vi "BMS.vi"() -> ()   [LabVIEW 2016]
panel:
  in  "node-ID":u8=1 min=1 max=127 step=1
  in  "baud rate":u32(ring) items=["1 Mbit/s"=0, "800 kbit/s"=1, "500 kbit/s"=2, "250 kbit/s"=3, "125 kbit/s"=4, "50 kbit/s"=6, "20 kbit/s"=7, "10 kbit/s"=8]
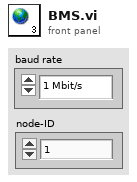
[diagram p1: front panel]
diagram:
